vi "FrequencyHelper.vi"(8 "error in (no error)":errorcluster) -> (0 "error out":errorcluster, 3 "List of Frequencies (Hz)":dbl[](array[numeric]))   [LabVIEW 2024]
panel:
  in  "Number of  Frequencies":i32=2 min=2
  in  "Stop Frequency":dbl
  in  "Generate List":bool
  in  "Start Frequency":dbl
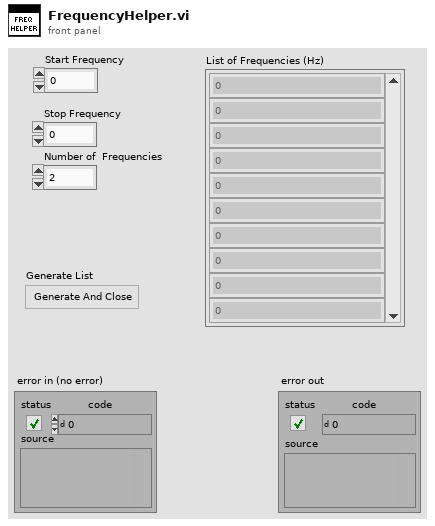
[diagram p1: front panel]
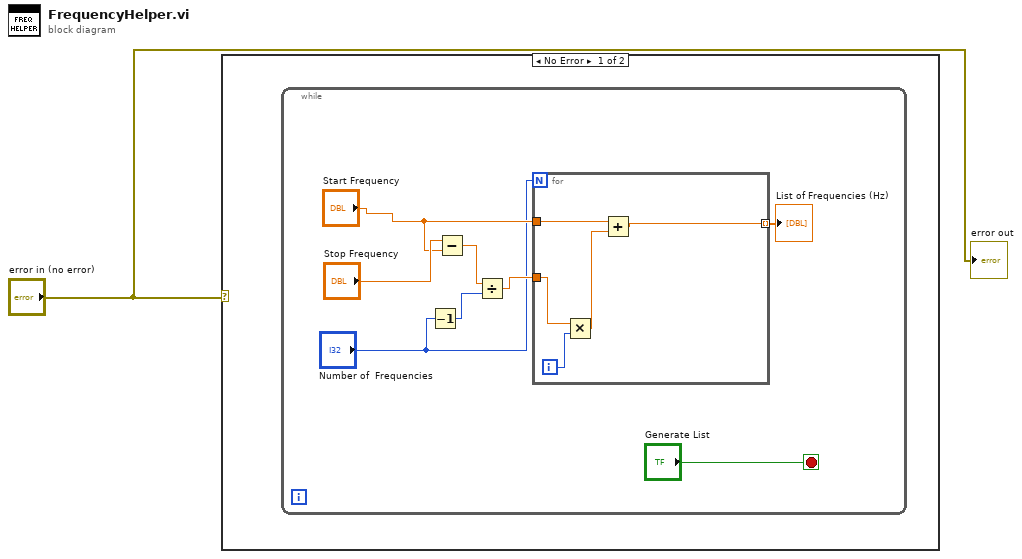
[diagram p0: block diagram]
diagram:
  n1 = case shown="No Error" "error in (no error)" {
    frame No Error {
      n2 = while {
        stop <- "Generate List" stop-if-true
        n3 = Decrement(x="Number of  Frequencies") -> (x-1=w2:i32)
        n4 = Subtract(x="Stop Frequency", y="Start Frequency") -> (x-y=w8:dbl)
        n5 = Divide(x=w8, y=w2) -> (x/y=w7:dbl)
        n6 = for {
          N: "Number of  Frequencies" -> [_]
          tunnel: "Start Frequency" -> [w14]
          tunnel: w7 -> [w12]
          tunnel: [w10] -> w6 mode=indexing
          i -> [w13]
          n7 = Multiply(x=w12, y=w13) -> (x*y=w11:dbl)
          n8 = Add(x=w14, y=w11) -> (x+y=w10:dbl)
        }
        "List of Frequencies (Hz)" <- w6
      }
    }
    frame Error {
    }
  }
  "error out" <- "error in (no error)"
